vi "仪器电源管理.vi"() -> ()   [LabVIEW 2016, in "环境动力监测库.lvlib" / "G电源管理库.lvlib"]
uses:
  <vilib>/Utility/miscctls.llb/LVPointTypeDef.ctl
panel:
  in  "电源控制":T1
  in  "副屏看门狗启用":u16(ring) caption="副屏看门狗启用：" items=["关闭", "打开"]
  in  "副屏看门狗设置":u16 caption="副屏看门狗设置："
  out "副屏看门狗计时":u16 caption="副屏看门狗计时："
  in  "主屏看门狗启用":u16(ring) caption="主屏看门狗启用：" items=["关闭", "打开"]
  in  "主屏看门狗设置":u16 caption="主屏看门狗设置："
  out "主屏看门狗计时":u16 caption="主屏看门狗计时："
  # "仪器电源管理"
  # "s"
  # "s"
  # "s"
  # "s"
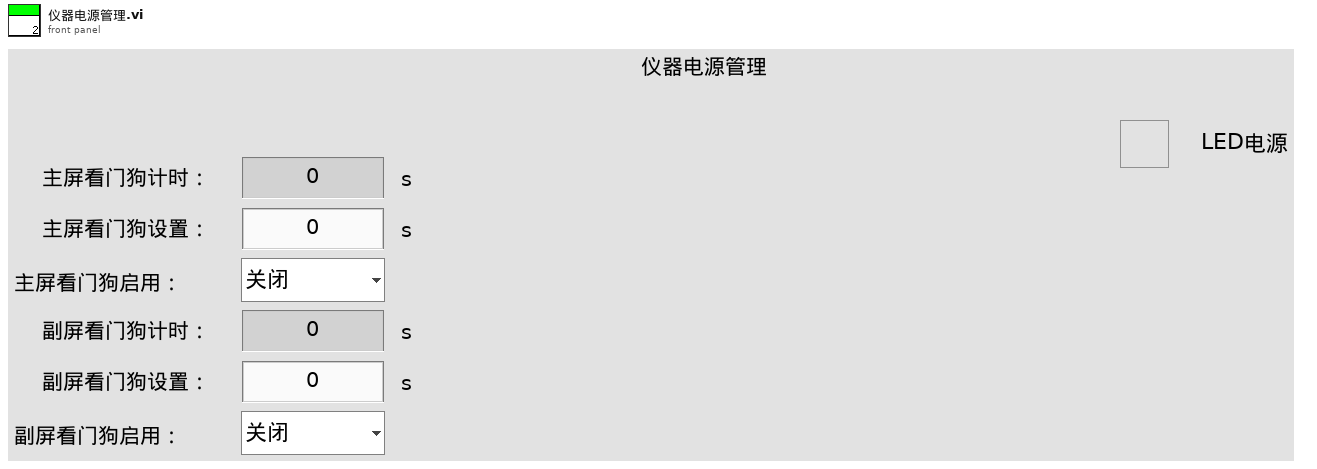
[diagram p1: front panel]
types:
  T1 = cluster{"氨氮电源":bool, "总磷电源":bool, "总氮电源":bool, "多参数电源":bool, "CODMn电源":bool, "CODCr电源":bool, "LED电源":bool}
  T2 = typedef "LVPointTypeDef.ctl" = cluster{"Horizontal":i16, "Vertical":i16}
  T3 = cluster{"采配水启用":bool, "CODMn启用":bool, "CODcr启用":bool, "氨氮启用":bool, "总磷启用":bool, "质控单元启用":bool, "流量计启用":bool, "电源管理启用":bool, "其他启用":bool, "多参数启用":bool, "超标留样启用":bool, "总氮启用":bool, "运行模式":enum16{"维护模式", "常规模式", "应急模式", "质控模式"}}
  T4 = cluster{"状态":cluster{"R0":i16, "R1":i16, "R2":i16, "R3":i16, "R4":i16, "R5":i16, "R6":i16, "R7":i16, "R8":i16, "R9":i16, "R10":i16, "R11":i16, "R12":i16, "R13":i16, "R14":i16, "R15":i16, "R16":i16, "R17":i16, "R18":i16, "R19":i16, "R20":i16, "R21":i16, "R22":i16, "R23":i16, "R24":i16, "R25":i16, "R26":i16, "R27":i16, "R28":i16, "R29":i16, "R30":i16, "R31":i16, "R32":i16, "R33":i16, "R34":i16, "R35":i16, "R36":i16, "R37":i16, "R38":i16, "R39":i16}, "输入状态":bool[], "输出状态":bool[], "参数设置":cluster{"R100":i16, "R101":i16, "R102":i16, "R103":i16, "R104":i16, "R105":i16, "R106":i16, "R107":i16, "R108":i16, "R109":i16, "R110":i16, "R111":i16, "R112":i16, "R113":i16, "R114":i16, "R115":i16, "R116":i16, "R117":i16, "R118":i16, "R119":i16, "R120":i16, "R121":i16, "R122":i16, "R123":i16}, "转换值":cluster{"AD0":sgl, "AD1":sgl, "AD2":sgl, "AD3":sgl, "AD4":sgl, "AD5":sgl}}
  T5 = cluster{"R0":i16, "R1":i16, "R2":i16, "R3":i16, "R4":i16, "R5":i16, "R6":i16, "R7":i16, "R8":i16, "R9":i16, "R10":i16, "R11":i16, "R12":i16, "R13":i16, "R14":i16, "R15":i16, "R16":i16, "R17":i16, "R18":i16, "R19":i16, "R20":i16, "R21":i16, "R22":i16, "R23":i16, "R24":i16, "R25":i16, "R26":i16, "R27":i16, "R28":i16, "R29":i16, "R30":i16, "R31":i16, "R32":i16, "R33":i16, "R34":i16, "R35":i16, "R36":i16, "R37":i16, "R38":i16, "R39":i16}
  T6 = cluster{"R100":i16, "R101":i16, "R102":i16, "R103":i16, "R104":i16, "R105":i16, "R106":i16, "R107":i16, "R108":i16, "R109":i16, "R110":i16, "R111":i16, "R112":i16, "R113":i16, "R114":i16, "R115":i16, "R116":i16, "R117":i16, "R118":i16, "R119":i16, "R120":i16, "R121":i16, "R122":i16, "R123":i16}
  T7 = cluster{"网络状态":bool, "电源管理":cluster{"电源管理":bool, "氨氮电源":bool, "总磷电源":bool, "总氮电源":bool, "多参数电源":bool, "CODMn电源":bool, "CODCr电源":bool, "灯带电源":bool, "照明电源":bool}, "北斗-GPS":cluster{"北斗":cluster{"经度:":sgl, "纬度:":sgl, "北斗监测":bool}, "GPS":cluster{"经度:":sgl, "纬度: ":sgl, "GPS监测":bool}}}
  T8 = cluster{"命令":string, "数据":cluster{"starting address":u16, "holding register values":u16[]}}
  T9 = cluster{"命令":string, "数据":cluster{"starting address":u16, "holding register value":u16}}
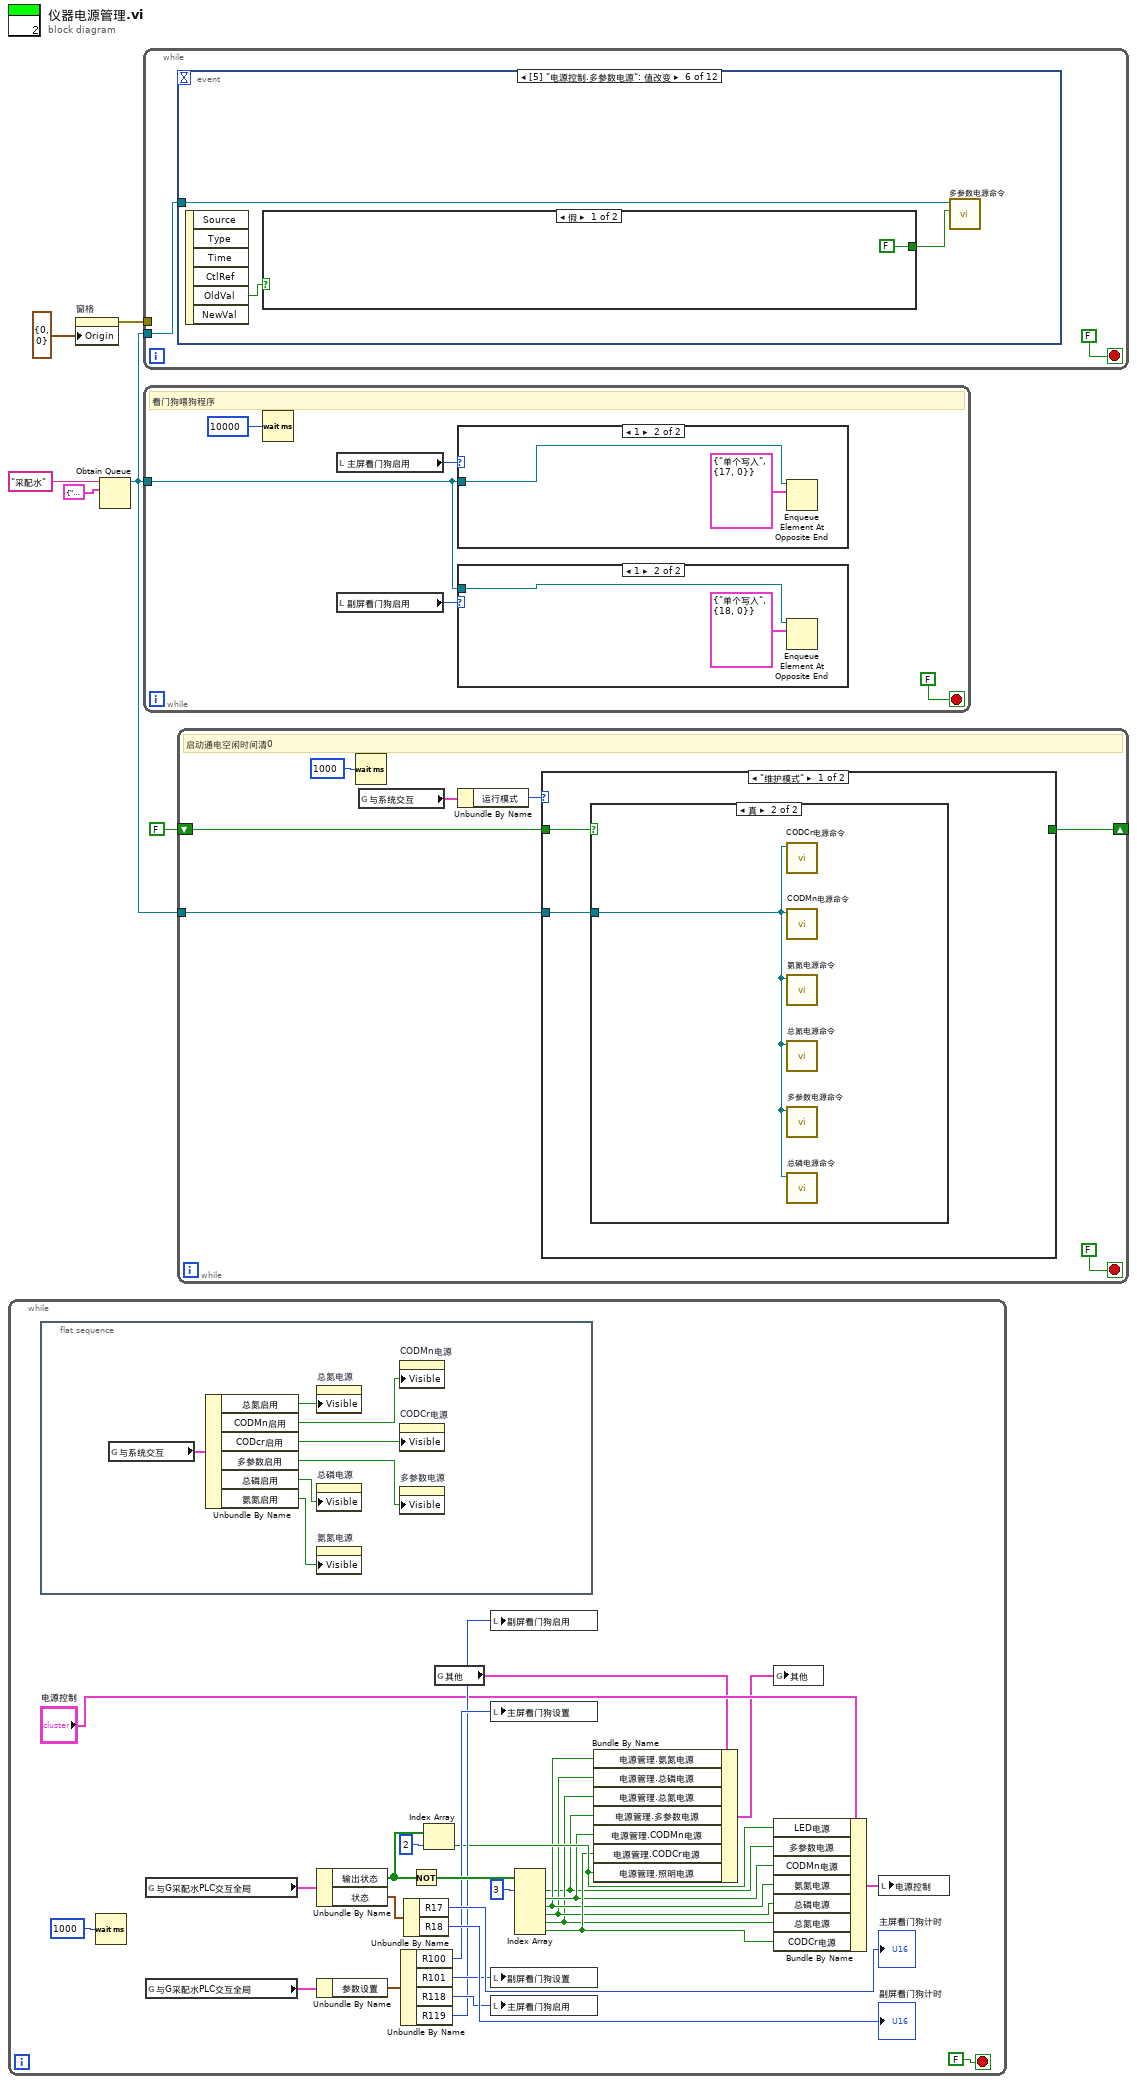
[diagram p0: block diagram]
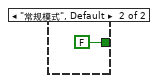
[diagram p5: hidden frame]
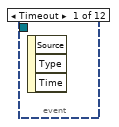
[diagram p6: hidden frame]
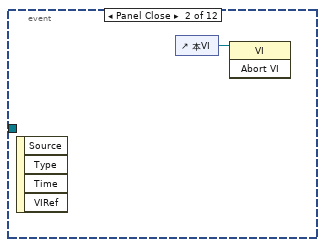
[diagram p7: hidden frame]
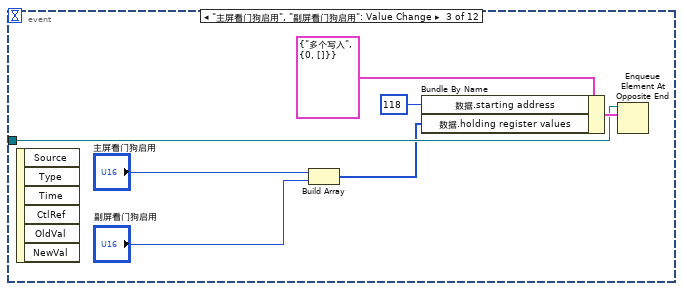
[diagram p8: hidden frame]
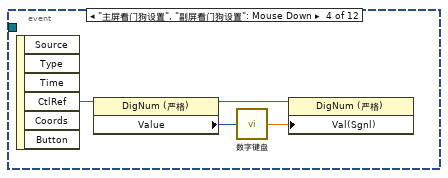
[diagram p9: hidden frame]
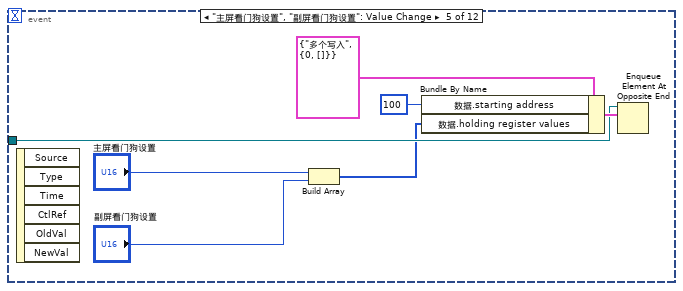
[diagram p10: hidden frame]
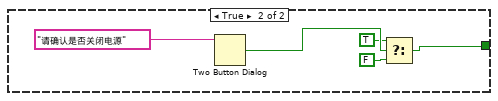
[diagram p11: hidden frame]
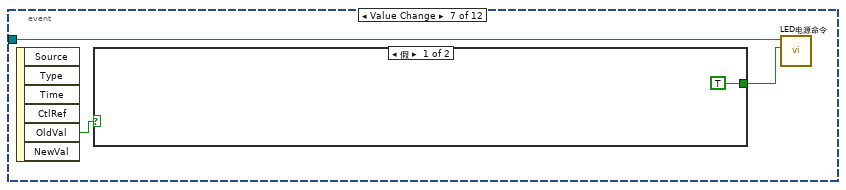
[diagram p12: hidden frame]
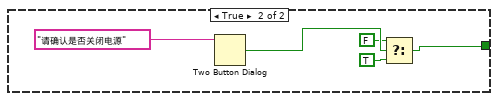
[diagram p13: hidden frame]
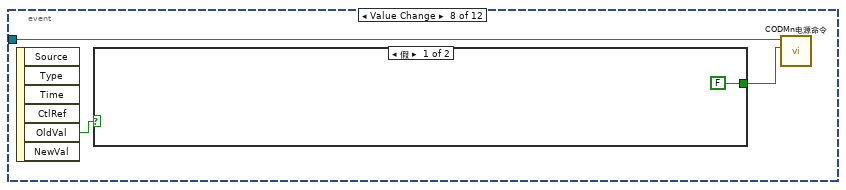
[diagram p14: hidden frame]
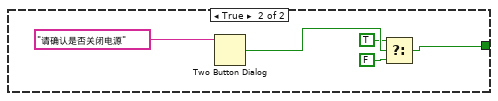
[diagram p15: hidden frame]
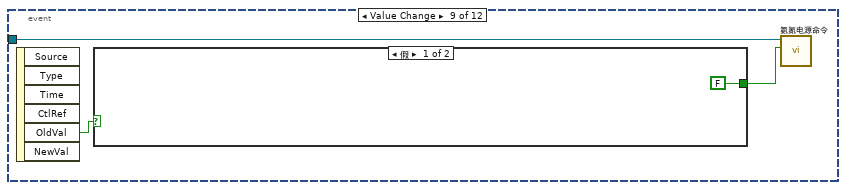
[diagram p16: hidden frame]
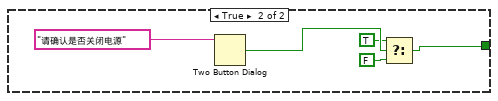
[diagram p17: hidden frame]
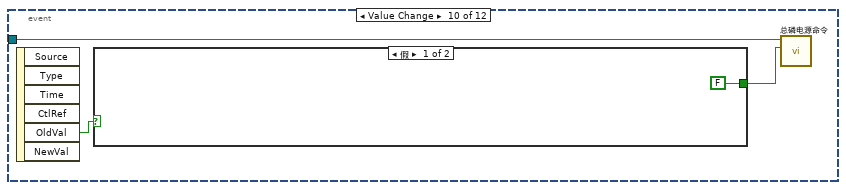
[diagram p18: hidden frame]
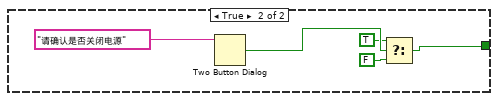
[diagram p19: hidden frame]
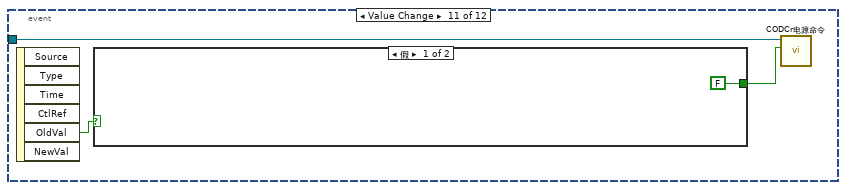
[diagram p20: hidden frame]
diagram:
  n1 = while {
    stop <- FALSE stop-if-true
    n2 = flat-sequence {
      frame #0 {
        n3 = global read "外部交互全局变量.vi" "与系统交互"() -> (w40:T3)
        n4 = Unbundle By Name(w40) -> ("总氮启用"=w39:bool, "CODMn启用"=w38:bool, "CODcr启用"=w34:bool, "多参数启用"=w35:bool, "总磷启用"=w36:bool, "氨氮启用"=w37:bool)
        n5 = property on="总氮电源" class="Bool (严格)"("Visible"=w39) -> ()  [unwired: 2 in, 2 out]
        n6 = property on="总磷电源" class="Bool (严格)"("Visible"=w36) -> ()  [unwired: 2 in, 2 out]
        n7 = property on="氨氮电源" class="Bool (严格)"("Visible"=w37) -> ()  [unwired: 2 in, 2 out]
        n8 = property on="CODMn电源" class="Bool (严格)"("Visible"=w38) -> ()  [unwired: 2 in, 2 out]
        n9 = property on="CODCr电源" class="Bool (严格)"("Visible"=w34) -> ()  [unwired: 2 in, 2 out]
        n10 = property on="多参数电源" class="Bool (严格)"("Visible"=w35) -> ()  [unwired: 2 in, 2 out]
      }
    }
    n11 = Wait (ms)(milliseconds to wait=u32 1000 ("等待时间（毫秒）")) -> ()  [unwired: 1 out]
    n12 = global read "外部交互全局变量.vi" "与G采配水PLC交互全局"() -> (w18:T4)
    n13 = global read "外部交互全局变量.vi" "与G采配水PLC交互全局"() -> (w20:T4)
    n14 = Unbundle By Name(w18) -> ("输出状态"=w17:bool[], "状态"=w16:T5)
    n15 = Unbundle By Name(w20) -> ("参数设置"=w19:T6)
    n16 = Unbundle By Name(w19) -> ("R100"=w28:i16, "R101"=w27:i16, "R118"=w26:i16, "R119"=w25:i16)
    n17 = Unbundle By Name(w16) -> ("R17"=→"主屏看门狗计时":i16, "R18"=→"副屏看门狗计时":i16)
    n18 = Not(x=w17) -> (.not. x?=w31:bool[])
    n19 = Index Array(array=w17, index=2 ("索引")) -> (element=w13:bool)
    n20 = global read "内部交互全局变量.vi" "其他"() -> (w14:T7)
    n21 = local write "副屏看门狗启用"(w25) -> ()
    n22 = local write "主屏看门狗设置"(w28) -> ()
    n23 = local write "副屏看门狗设置"(w27) -> ()
    n24 = local write "主屏看门狗启用"(w26) -> ()
    n25 = Index Array(array=w31, index #1=3 ("索引")) -> (element #1=w7:bool, element #2=w11:bool, element #3=w10:bool, element #4=w9:bool, element #5=w8:bool, element #6=w12:bool)  [unwired: 5 in]
    n26 = Bundle By Name(cluster=w14, "电源管理.氨氮电源"=w10, "电源管理.总磷电源"=w9, "电源管理.总氮电源"=w8, "电源管理.多参数电源"=w7, "电源管理.CODMn电源"=w11, "电源管理.CODCr电源"=w12, "电源管理.照明电源"=w13) -> (w15:T7)
    n27 = global write "内部交互全局变量.vi" "其他"(w15) -> ()
    n28 = Bundle By Name(cluster="电源控制", "LED电源"=w13, "多参数电源"=w7, "CODMn电源"=w11, "氨氮电源"=w10, "总磷电源"=w9, "总氮电源"=w8, "CODCr电源"=w12) -> (w21:T1)
    n29 = local write "电源控制"(w21) -> ()
  }
  n30 = property on="窗格" class="Pane"("Origin"=T2 {"Horizontal"=0, "Vertical"=0} ("原点")) -> (error out=w3:errorcluster)  [unwired: 2 in, 1 out]
  n31 = Obtain Queue(name (unnamed)="采配水" ("名称（未命名）"), element data type=cluster{"命令":string, "数据":variant} {"命令"="", "数据"=variant}) -> (queue out=w1:refnum<queue>)  [unwired: 3 in, 2 out]
  n32 = while {
    tunnel: w1 -> [w42]
    tunnel: w3 -> [_]
    stop <- FALSE stop-if-true
    n33 = event shown="[5] \"电源控制.多参数电源\": 值改变" {
      selector: _ -> [_ _ _ _ _ _ _ _ _ _ _ _]
      dyn-events: _ -> [_ _ _ _ _ _ _ _ _ _ _ _]
      timeout: _ -> [_ _ _ _ _ _ _ _ _ _ _ _]
      tunnel: w42 -> [_ _ w47 _ w58 w64 w72 w82 w91 w100 w109 w118]
      event Timeout {
        n34 = event-data() -> ()  [unwired: 1 in, 3 out]
      }
      event Panel Close {
        n35 = event-data() -> ()  [unwired: 1 in, 4 out]
        n36 = control-ref of="本VI"() -> (w43:refnum<vi>)
        n37 = invoke class="VI" method="Abort VI"(reference=w43) -> ()  [unwired: 2 in, 3 out]
      }
      event "主屏看门狗启用", "副屏看门狗启用": Value Change {
        n38 = event-data() -> ()  [unwired: 1 in, 6 out]
        n39 = Build Array("主屏看门狗启用", "副屏看门狗启用") -> (w44:u16[])
        n40 = Bundle By Name(cluster=T8 {"命令"="多个写入", "数据"={"starting address"=0, "holding register values"=[]}} ("元素"), "数据.starting address"=u16 118, "数据.holding register values"=w44) -> (w48:T8)
        n41 = Enqueue Element At Opposite End(queue=w47, element=w48) -> ()  [unwired: 2 in, 3 out]
      }
      event "主屏看门狗设置", "副屏看门狗设置": Mouse Down {
        n42 = event-data() -> ("CtlRef"=w51:refnum<vi>)  [unwired: 1 in, 5 out]
        n43 = property class="DigNum (严格)"(reference=w51) -> (reference out=w53:refnum<vi>, "Value"=w54:u16)  [unwired: 1 in, 1 out]
        n44 = call "数字键盘.vi"("OldNumber"=w54) -> ("NewNumber"=w52:sgl)
        n45 = property class="DigNum (严格)"(reference=w53, "Val(Sgnl)"=w52) -> ()  [unwired: 1 in, 2 out]
      }
      event "主屏看门狗设置", "副屏看门狗设置": Value Change {
        n46 = event-data() -> ()  [unwired: 1 in, 6 out]
        n47 = Build Array("主屏看门狗设置", "副屏看门狗设置") -> (w55:u16[])
        n48 = Bundle By Name(cluster=T8 {"命令"="多个写入", "数据"={"starting address"=0, "holding register values"=[]}} ("元素"), "数据.starting address"=u16 100, "数据.holding register values"=w55) -> (w59:T8)
        n49 = Enqueue Element At Opposite End(queue=w58, element=w59) -> ()  [unwired: 2 in, 3 out]
      }
      event "电源控制.多参数电源": Value Change {
        n50 = event-data() -> ("OldVal"=w63:bool)  [unwired: 1 in, 5 out]
        n51 = case shown="假" w63 {
          tunnel: [FALSE ("T button?") w66] -> w62
          frame False {
          }
          frame True {
            n52 = Two Button Dialog(message="请确认是否关闭电源" ("消息")) -> (T button?=w69:bool)  [unwired: 2 in]
            n53 = Select(t=TRUE, s=w69, f=FALSE ("T button?")) -> (s? t:f=w66:bool)
          }
        }
        n54 = call "多参数电源命令.vi"("通电/断电"=w62, "队列"=w64) -> ()  [unwired: 9 in, 1 out]
      }
      event "电源控制.LED电源": Value Change {
        n55 = event-data() -> ("OldVal"=w73:bool)  [unwired: 1 in, 5 out]
        n56 = case shown="假" w73 {
          tunnel: [TRUE ("T button?") w75] -> w71
          frame False {
          }
          frame True {
            n57 = Two Button Dialog(message="请确认是否关闭电源" ("消息")) -> (T button?=w78:bool)  [unwired: 2 in]
            n58 = Select(t=FALSE, s=w78, f=TRUE ("T button?")) -> (s? t:f=w75:bool)
          }
        }
        n59 = call "LED电源命令.vi"("通电/断电"=w71, "队列"=w72) -> ()  [unwired: 9 in, 1 out]
      }
      event "电源控制.CODMn电源": Value Change {
        n60 = event-data() -> ("OldVal"=w81:bool)  [unwired: 1 in, 5 out]
        n61 = case shown="假" w81 {
          tunnel: [FALSE ("T button?") w84] -> w80
          frame False {
          }
          frame True {
            n62 = Two Button Dialog(message="请确认是否关闭电源" ("消息")) -> (T button?=w87:bool)  [unwired: 2 in]
            n63 = Select(t=TRUE, s=w87, f=FALSE ("T button?")) -> (s? t:f=w84:bool)
          }
        }
        n64 = call "CODMn电源命令.vi"("通电/断电"=w80, "队列"=w82) -> ()  [unwired: 9 in, 1 out]
      }
      event "电源控制.氨氮电源": Value Change {
        n65 = event-data() -> ("OldVal"=w90:bool)  [unwired: 1 in, 5 out]
        n66 = case shown="假" w90 {
          tunnel: [FALSE ("T button?") w93] -> w89
          frame False {
          }
          frame True {
            n67 = Two Button Dialog(message="请确认是否关闭电源" ("消息")) -> (T button?=w96:bool)  [unwired: 2 in]
            n68 = Select(t=TRUE, s=w96, f=FALSE ("T button?")) -> (s? t:f=w93:bool)
          }
        }
        n69 = call "氨氮电源命令.vi"("通电/断电"=w89, "队列"=w91) -> ()  [unwired: 9 in, 1 out]
      }
      event "电源控制.总磷电源": Value Change {
        n70 = event-data() -> ("OldVal"=w99:bool)  [unwired: 1 in, 5 out]
        n71 = case shown="假" w99 {
          tunnel: [FALSE ("T button?") w102] -> w98
          frame False {
          }
          frame True {
            n72 = Two Button Dialog(message="请确认是否关闭电源" ("消息")) -> (T button?=w105:bool)  [unwired: 2 in]
            n73 = Select(t=TRUE, s=w105, f=FALSE ("T button?")) -> (s? t:f=w102:bool)
          }
        }
        n74 = call "总磷电源命令.vi"("通电/断电"=w98, "队列"=w100) -> ()  [unwired: 9 in, 1 out]
      }
      event "电源控制.CODCr电源": Value Change {
        n75 = event-data() -> ("OldVal"=w108:bool)  [unwired: 1 in, 5 out]
        n76 = case shown="假" w108 {
          tunnel: [FALSE ("T button?") w111] -> w107
          frame False {
          }
          frame True {
            n77 = Two Button Dialog(message="请确认是否关闭电源" ("消息")) -> (T button?=w114:bool)  [unwired: 2 in]
            n78 = Select(t=TRUE, s=w114, f=FALSE ("T button?")) -> (s? t:f=w111:bool)
          }
        }
        n79 = call "CODCr电源命令.vi"("通电/断电"=w107, "队列"=w109) -> ()  [unwired: 9 in, 1 out]
      }
      event "电源控制.总氮电源": Value Change {
        n80 = event-data() -> ("OldVal"=w116:bool)  [unwired: 1 in, 5 out]
        n81 = case shown="假" w116 {
          tunnel: [FALSE ("T button?") w120] -> w117
          frame False {
          }
          frame True {
            n82 = Two Button Dialog(message="请确认是否关闭电源" ("消息")) -> (T button?=w123:bool)  [unwired: 2 in]
            n83 = Select(t=TRUE, s=w123, f=FALSE ("T button?")) -> (s? t:f=w120:bool)
          }
        }
        n84 = call "总氮电源命令.vi"("通电/断电"=w117, "队列"=w118) -> ()  [unwired: 9 in, 1 out]
      }
    }
  }
  n85 = while {
    tunnel: w1 -> [w129]
    stop <- FALSE stop-if-true
    # "看门狗喂狗程序"
    n86 = Wait (ms)(milliseconds to wait=u32 10000 ("等待时间（毫秒）")) -> ()  [unwired: 1 out]
    n87 = local read "主屏看门狗启用"() -> (w128:u16)
    n88 = local read "副屏看门狗启用"() -> (w127:u16)
    n89 = case shown="1" w128 {
      tunnel: w129 -> [_ w132]
      frame 0, Default {
      }
      frame 1 {
        n90 = Enqueue Element At Opposite End(queue=w132, element=T9 {"命令"="单个写入", "数据"={"starting address"=17, "holding register value"=0}} ("元素")) -> ()  [unwired: 2 in, 3 out]
      }
    }
    n91 = case shown="1" w127 {
      tunnel: w129 -> [_ w130]
      frame 0, Default {
      }
      frame 1 {
        n92 = Enqueue Element At Opposite End(queue=w130, element=T9 {"命令"="单个写入", "数据"={"starting address"=18, "holding register value"=0}} ("元素")) -> ()  [unwired: 2 in, 3 out]
      }
    }
  }
  n93 = while {
    tunnel: w1 -> [w138]
    shift-right: [w136] -> _
    shift-left: FALSE -> [w137]
    stop <- FALSE stop-if-true
    # "启动通电空闲时间清0"
    n94 = Wait (ms)(milliseconds to wait=u32 1000 ("等待时间（毫秒）")) -> ()  [unwired: 1 out]
    n95 = global read "外部交互全局变量.vi" "与系统交互"() -> (w135:T3)
    n96 = Unbundle By Name(w135) -> ("运行模式"=w134:enum16{"维护模式", "常规模式", "应急模式", "质控模式"})
    n97 = case shown="\"维护模式\"" w134 {
      tunnel: w138 -> [w142 _]
      tunnel: w137 -> [w141 _]
      tunnel: [_ FALSE] -> w136
      frame "维护模式" {
        n98 = case shown="真" w141 {
          tunnel: w142 -> [_ w143]
          frame False {
          }
          frame True {
            n99 = call "CODCr电源命令.vi"("队列"=w143) -> ()  [unwired: 10 in, 1 out]
            n100 = call "CODMn电源命令.vi"("队列"=w143) -> ()  [unwired: 10 in, 1 out]
            n101 = call "氨氮电源命令.vi"("队列"=w143) -> ()  [unwired: 10 in, 1 out]
            n102 = call "总氮电源命令.vi"("队列"=w143) -> ()  [unwired: 10 in, 1 out]
            n103 = call "多参数电源命令.vi"("队列"=w143) -> ()  [unwired: 10 in, 1 out]
            n104 = call "总磷电源命令.vi"("队列"=w143) -> ()  [unwired: 10 in, 1 out]
          }
        }
      }
      frame "常规模式", Default {
      }
    }
  }
